vi "Create Point by Size.vi"(8 "error in (no error)":errorcluster caption="错误输入（无错误）", 11 "Size.lvclass":refnum<class "Size.lvclass">) -> (0 "error out":errorcluster caption="错误输出", 3 "Point 输出":refnum<class "Point.lvclass"> caption="DNL_LabVIEW Object out")   [LabVIEW 2011, in "Point.lvclass"]
uses:
  Point.lvclass
  Size/Size.lvclass
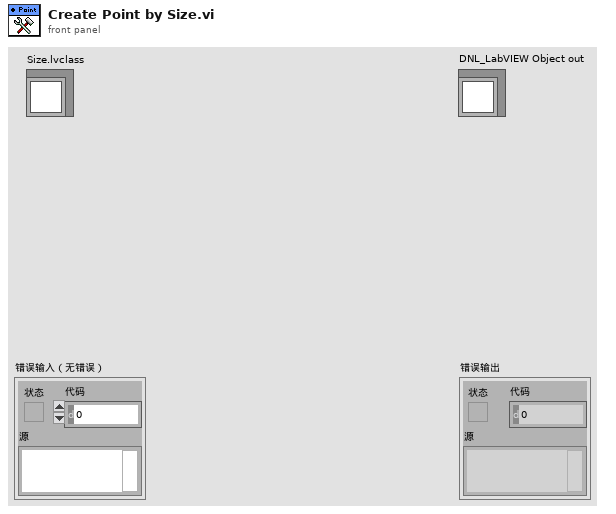
[diagram p1: front panel]
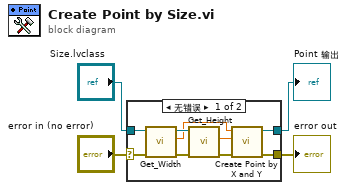
[diagram p0: block diagram]
diagram:
  n1 = case shown="无错误" "error in (no error)" {
    selector: "error in (no error)" -> [w6 w14]
    tunnel: [w5 w14] -> w3
    tunnel: "Size.lvclass" -> [w13 _]
    tunnel: [w7 _] -> w1
    frame No Error {
      n2 = call "Get_Width.vi"("error in (no error)"=w6, "Size输入"=w13) -> ("error out"=w9:errorcluster, "Width"=w11:dbl, "Size输出"=w12:refnum<class "Size.lvclass">)  [unwired: 7 in]
      n3 = call "Get_Height.vi"("error in (no error)"=w9, "Size输入"=w12) -> ("error out"=w8:errorcluster, "Height"=w10:dbl)  [unwired: 7 in, 1 out]
      n4 = call "Create Point by X and Y.vi"("error in (no error)"=w8, "Y"=w10, "X"=w11) -> ("error out"=w5:errorcluster, "Point 输出"=w7:refnum<class "Point.lvclass">)  [unwired: 7 in]
    }
    frame Error {
    }
  }
  "error out" <- w3
  "Point 输出" <- w1
